vi "Initialize.vi"(7 "Serial Configuration":T1={"Baud Rate"=9600, "Parity"=0, "Data Bits"=8, "Stop Bits"=10, "Flow Control"=2} {"Flow Control" items=["None", "XON/XOFF", "RTS/CTS", "XON/XOFF & RTS/CTS", "DTR/DSR", "XON/XOFF & DTR/DSR"]; "Stop Bits" items=["1.0"=10, "1.5"=15, "2.0"=20]; "Data Bits" items=["7"=7, "8"=8]; "Parity" items=["None", "Odd", "Even", "Mark", "Space"]; "Baud Rate" items=["300"=300, "600"=600, "1200"=1200, "2400"=2400, "4800"=4800, "9600"=9600, "19200"=19200]}, 8 "error in (no error)":errorcluster, 9 "Reset (True)":bool=TRUE, 10 "ID Query (True)":bool=TRUE, 11 "VISA resource name":refnum<visa-resource-name>) -> (0 "error out":errorcluster, 3 "VISA resource name out":refnum<visa-resource-name>)   [LabVIEW 2020, in "Stanford Research DG645.lvlib"]
doc: "Establishes communication with the instrument and optionally performs an instrument identification query and/or an instrument reset. It also places the instrument in a default state needed for other instrument driver operations. Therefore, call this VI before calling other instrument driver VIs for this instrument. Generally, you need to call the <B>Initialize</B> VI only once at the beginning of an application."
uses:
  Downloads/stanford_research_dg645/Stanford Research DG645/Stanford Research DG645.lvlib
panel:
  # "(c) 2013 National Instruments Corp.  ALL RIGHTS RESERVED."
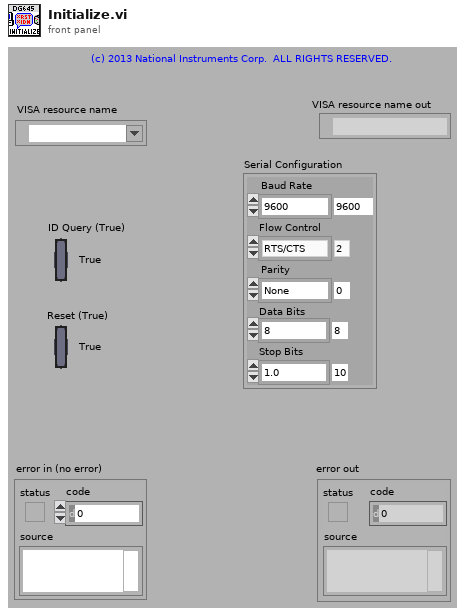
[diagram p1: front panel]
types:
  T1 = cluster{"Baud Rate":u32, "Parity":u16, "Data Bits":u16, "Stop Bits":u16, "Flow Control":u16}
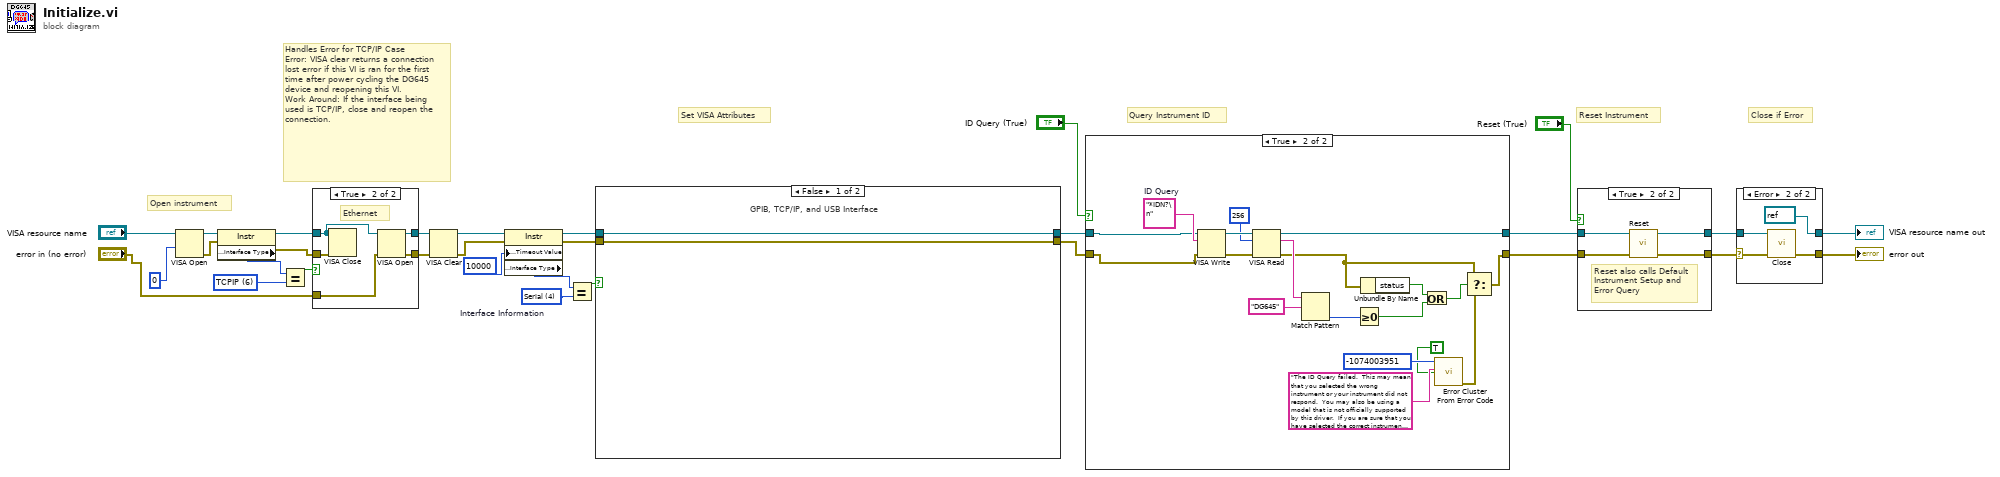
[diagram p0: block diagram]
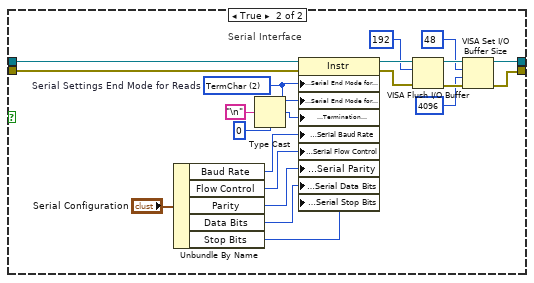
[diagram p3: hidden frame]
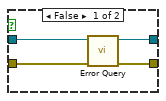
[diagram p5: hidden frame]
diagram:
  w8 = u16 6 items=["GPIB"=1, "VXI"=2, "GPIB-VXI"=3, "Serial"=4, "PXI"=5, "TCPIP"=6, "USB"=7] ("Interface Information:Interface Type")
  w19 = u16 4 items=["GPIB"=1, "VXI"=2, "GPIB-VXI"=3, "Serial"=4, "PXI"=5, "TCPIP"=6, "USB"=7]  # Interface Information
  # "Handles Error for TCP/IP Case\nError: VISA clear returns a connection lost error if this VI is ran for the first time after power cycling the DG645 device and reopening this VI.\nWork Around: If the interface being used is TCP/IP, close and reopen the connection."
  # "Set VISA Attributes"
  # "Close if Error"
  # "Query Instrument ID"
  # "Reset Instrument"
  # "Open instrument"
  n1 = VISA Open(access mode=u32 0, VISA resource name="VISA resource name") -> (VISA resource name=w10:refnum<visa-resource-name>, error out=w4:errorcluster)  [unwired: 3 in]
  n2 = property on="Property Node" class="Instr"(reference=w10, error in=w4) -> (reference out=w5:refnum<visa-resource-name>, error out=w6:errorcluster, "Interface Information:Interface Type"=w7:u16)
  n3 = Equal?(x=w7, y=w8) -> (x = y?=w9:bool)
  n4 = case shown="True" w9 {
    tunnel: [w31 w37] -> w11
    tunnel: w6 -> [w32 w36]
    tunnel: w5 -> [w31 w35]
    tunnel: [w32 w33] -> w3
    tunnel: "error in (no error)" -> [_ w34]
    frame False {
      # "GPIB\nSerial"
    }
    frame True {
      # "Ethernet"
      n5 = VISA Close(VISA resource name=w35, error in (no error)=w36) -> ()  [unwired: 1 out]
      n6 = VISA Open(error in (no error)=w34, VISA resource name=w35) -> (VISA resource name=w37:refnum<visa-resource-name>, error out=w33:errorcluster)  [unwired: 3 in]
    }
  }
  n7 = VISA Clear(VISA resource name=w11, error in (no error)=w3) -> (VISA resource name out=w12:refnum<visa-resource-name>, error out=w13:errorcluster)
  n8 = property on="Property Node" class="Instr"(reference=w12, error in=w13, "General Settings:Timeout Value"=u32 10000) -> (reference out=w22:refnum<visa-resource-name>, error out=w21:errorcluster, "Interface Information:Interface Type"=w26:u16)
  n9 = Equal?(x=w26, y=w19) -> (x = y?=w20:bool)
  n10 = case shown="False" w20 {
    tunnel: [w38 w57] -> w24
    tunnel: [w39 w54] -> w23
    tunnel: w22 -> [w38 w59]
    tunnel: w21 -> [w39 w60]
    frame False {
      # "GPIB, TCP/IP, and USB Interface"
    }
    frame True {
      w47 = u16 2 items=["None", "LastBit", "TermChar"]  # Serial Settings End Mode for Reads
      # "Serial Interface"
      n11 = Unbundle By Name("Serial Configuration") -> ("Baud Rate"=w45:u32, "Flow Control"=w41:u16, "Parity"=w43:u16, "Data Bits"=w44:u16, "Stop Bits"=w40:u16)
      n12 = Type Cast(type=u8 0, x="\n" ("Line Feed Constant")) -> (*(type *) &x=w46:u8)
      n13 = property on="Property Node" class="Instr"(reference=w59, error in=w60, "Serial Settings:Serial End Mode for Reads"=w47, "Serial Settings:Serial End Mode for Writes"=w47, "Message Based Settings:Termination Character"=w46, "Serial Settings:Serial Baud Rate"=w45, "Serial Settings:Serial Flow Control"=w41, "Serial Settings:Serial Parity"=w43, "Serial Settings:Serial Data Bits"=w44, "Serial Settings:Serial Stop Bits"=w40) -> (reference out=w53:refnum<visa-resource-name>, error out=w56:errorcluster)
      n14 = VISA Flush I/O Buffer(VISA resource name=w53, mask (16)=u16 192, error in (no error)=w56) -> (VISA resource name out=w58:refnum<visa-resource-name>, error out=w55:errorcluster)
      n15 = VISA Set I/O Buffer Size(VISA resource name=w58, mask (16)=u16 48, size (4096)=u32 4096 ("size (0)"), error in (no error)=w55) -> (VISA resource name out=w57:refnum<visa-resource-name>, error out=w54:errorcluster)
    }
  }
  n16 = case shown="True" "ID Query (True)" {
    tunnel: [w61 w81] -> w29
    tunnel: [w62 w80] -> w30
    tunnel: w24 -> [w62 w64]
    tunnel: w23 -> [w61 w63]
    frame False {
    }
    frame True {
      w74 = "*IDN?\n"  # ID Query
      n17 = VISA Write(VISA resource name=w64, write buffer=w74, error in (no error)=w63) -> (VISA resource name out=w78:refnum<visa-resource-name>, error out=w77:errorcluster)  [unwired: 1 out]
      n18 = VISA Read(VISA resource name=w78, byte count=u32 256, error in (no error)=w77) -> (VISA resource name out=w80:refnum<visa-resource-name>, read buffer=w79:string, error out=w68:errorcluster)  [unwired: 1 out]
      n19 = Match Pattern(string=w79, regular expression="DG645") -> (offset past match=w69:i32)  [unwired: 1 in, 3 out]
      n20 = Greater Or Equal To 0?(x=w69) -> (x >= 0?=w66:bool)
      n21 = Unbundle By Name(w68) -> ("status"=w67:bool)
      n22 = Or(x=w67, y=w66) -> (x .or. y?=w65:bool)
      n23 = call <vilib>:"Error Cluster From Error Code.vi"("show call chain? (False)"=TRUE, "error message (\"\")"="The ID Query failed.  This may mean that you selected the wrong instrument or your instrument did not respond.  You may also be using a model that is not officially supported by this driver.  If you are sure that you have selected the correct instrument and it is responding, try disabling the ID Query." ("Source (VI Name)"), "error code (0)"=-1074003951 ("Code")) -> ("error out"=w73:errorcluster)  [unwired: 6 in]
      n24 = Select(t=w68, s=w65, f=w73) -> (s? t:f=w81:errorcluster)
    }
  }
  n25 = case shown="True" "Reset (True)" {
    tunnel: w29 -> [w82 w86]
    tunnel: [w84 w89] -> w14
    tunnel: w30 -> [w83 w87]
    tunnel: [w85 w88] -> w15
    frame False {
      n26 = call "Error Query.vi"("error in (no error)"=w82, "VISA resource name"=w83) -> ("error out"=w84:errorcluster, "VISA resource name out"=w85:refnum<visa-resource-name>)  [unwired: 6 in, 2 out]
    }
    frame True {
      # "Reset also calls Default Instrument Setup and Error Query"
      n27 = call "Reset.vi"("error in (no error)"=w86, "VISA resource name"=w87) -> ("error out"=w89:errorcluster, "VISA resource name out"=w88:refnum<visa-resource-name>)  [unwired: 8 in]
    }
  }
  n28 = case shown="Error" w14 {
    selector: w14 -> [w90 w93]
    tunnel: w15 -> [w91 w94]
    tunnel: [w91 refnum<visa-resource-name> refnum ("VISA resource name out")] -> w17
    tunnel: [w90 w95] -> w16
    frame No Error {
    }
    frame Error {
      n29 = call "Close.vi"("error in (no error)"=w93, "VISA resource name"=w94) -> ("error out"=w95:errorcluster)  [unwired: 9 in]
    }
  }
  "VISA resource name out" <- w17
  "error out" <- w16
